vi "reshapeArray_FGV.vi"(4 "delete":dbl[](array[numeric])=[0.0, -1800.0, 0.0], 6 "firstpixelpos":dbl[](array[numeric]), 7 "command":T1=enum."read", 8 "error in (no error)":errorcluster, 9 "reshapedArray CamX":dbl[](array[numeric]), 10 "index":i32, 11 "emptyImageArray":dbl[](array[numeric])) -> (0 "error in (no error) 2":errorcluster, 3 "ImageArray":dbl[](array[numeric]))   [LabVIEW 2020]
uses:
  reshapeArrayCommand_TypDEf.ctl
panel:
  out "index 3":dbl
  out "del2 3":dbl
  out "del1 3":dbl
  out "size(s) 3":i32
  out "index 2":dbl
  out "del2 2":dbl
  out "del1 2":dbl
  out "size(s) 2":i32
  out "index":dbl
  out "Array":dbl[](array[numeric])
  in  "y":i32
  out "del2":dbl
  out "del1":dbl
  out "size(s)":i32
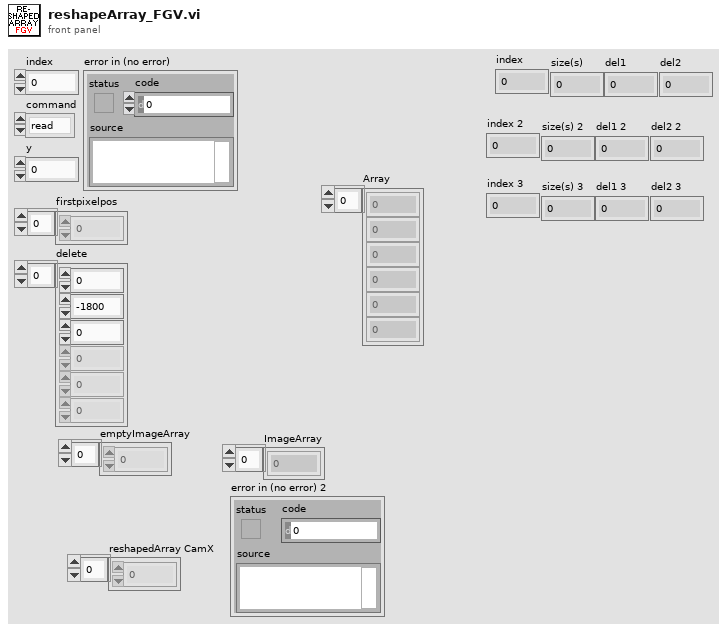
[diagram p1: front panel]
types:
  T1 = typedef "reshapeArrayCommand_TypDEf.ctl" = enum16{"init array", "addImage", "read", "init resolution"}
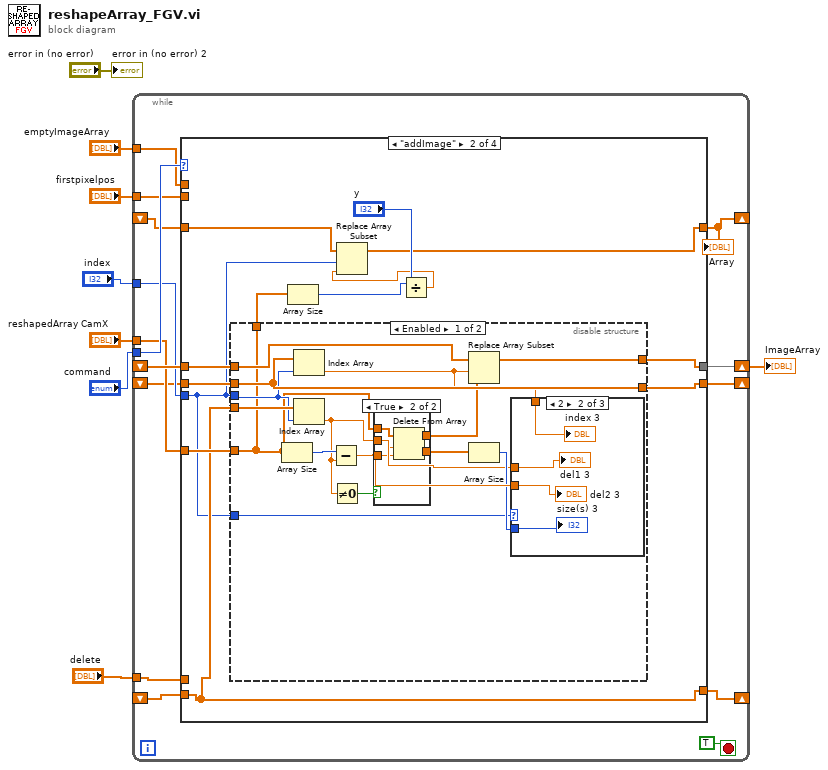
[diagram p0: block diagram]
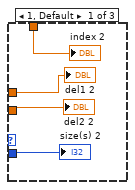
[diagram p4: hidden frame]
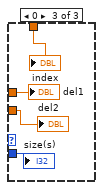
[diagram p5: hidden frame]
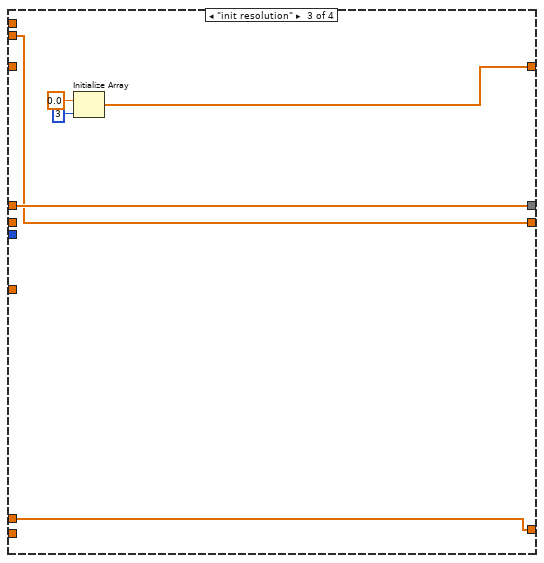
[diagram p7: hidden frame]
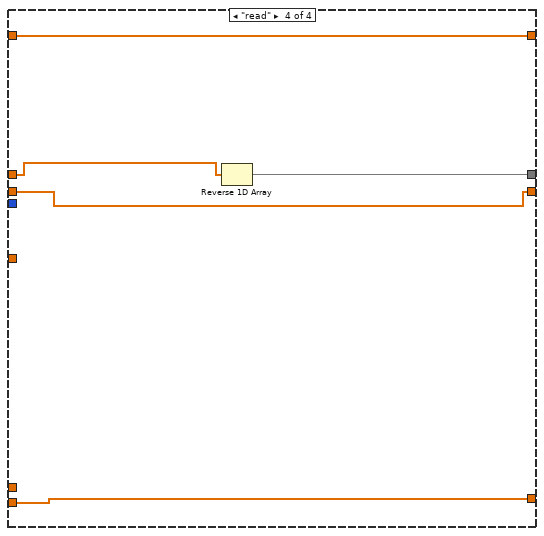
[diagram p8: hidden frame]
diagram:
  n1 = while {
    tunnel: "command" -> [w23]
    tunnel: "emptyImageArray" -> [w22]
    shift-right: [w21] -> w1
    shift-left: _ -> [w20]
    tunnel: "reshapedArray CamX" -> [w18]
    tunnel: "index" -> [w19]
    tunnel: "firstpixelpos" -> [w17]
    shift-right: [w15] -> _
    shift-left: _ -> [w14]
    tunnel: "delete" -> [w13]
    shift-right: [w12] -> _
    shift-left: _ -> [w11]
    shift-right: [w10] -> _
    shift-left: _ -> [w9]
    stop <- TRUE stop-if-true
    n2 = case shown="\"addImage\"" w23 {
      tunnel: w22 -> [w27 _ _ _]
      tunnel: [w27 w37 w79 w83] -> w21
      tunnel: w20 -> [_ w40 w79 w81]
      tunnel: w19 -> [_ w28 _ _]
      tunnel: w18 -> [_ w39 _ _]
      tunnel: w17 -> [_ _ w78 _]
      tunnel: [w26 w36 w78 w84] -> w15
      tunnel: w14 -> [w26 w38 _ w84]
      tunnel: w13 -> [_ _ w77 _]
      tunnel: [w25 w35 w77 w82] -> w12
      tunnel: w11 -> [w25 w35 _ w82]
      tunnel: [w24 w29 w74 w80] -> w10
      tunnel: w9 -> [w24 w30 _ w80]
      frame "init array", Default {
      }
      frame "addImage" {
        n3 = disable-structure shown="Enabled" {
          disable-tunnel: w40 -> [w51 _]
          disable-tunnel: w39 -> [w44 _]
          disable-tunnel: w28 -> [w52 _]
          disable-tunnel: w38 -> [w54 _]
          disable-tunnel: [w55 _] -> w37
          disable-tunnel: [w54 _] -> w36
          disable-tunnel: w35 -> [w53 _]
          disable-tunnel: [w44 _] -> w34
          disable-tunnel: w28 -> [w41 _]
          frame Enabled {
            n4 = Array Size(array=w44) -> (size(s)=w48:i32)
            n5 = Index Array(array=w54, index=w52) -> (element=w42:dbl)
            n6 = Index Array(array=w53, index=w52) -> (element=w43:dbl)
            n7 = Subtract(x=w48, y=w43) -> (x-y=w47:dbl)
            n8 = Not Equal To 0?(x=w43) -> (x != 0?=w45:bool)
            n9 = case shown="True" w45 {
              tunnel: [w56 w61] -> w50
              tunnel: [_ w60] -> w49
              tunnel: w44 -> [w56 w59]
              tunnel: w43 -> [_ w58]
              tunnel: w47 -> [_ w57]
              frame False {
              }
              frame True {
                n10 = Delete From Array(array=w59, length=w58, index=w57) -> (deleted portion=w60:dbl[], array with subset deleted=w61:dbl[])
              }
            }
            n11 = Replace Array Subset(array=w51, new element=w50, index=w42) -> (w55:dbl[])
            n12 = Array Size(array=w49) -> (size(s)=w46:i32)
            n13 = case shown="2" w41 {
              tunnel: w46 -> [w62 w69 w73]
              tunnel: w43 -> [w64 w67 w72]
              tunnel: w47 -> [w63 w68 w71]
              tunnel: w42 -> [w65 w66 w70]
              frame 1, Default {
                "del2 2" <- w63
                "del1 2" <- w64
                "index 2" <- w65
                "size(s) 2" <- w62
              }
              frame 2 {
                "del2 3" <- w68
                "del1 3" <- w67
                "index 3" <- w66
                "size(s) 3" <- w69
              }
              frame 0 {
                "size(s)" <- w73
                "del1" <- w72
                "del2" <- w71
                "index" <- w70
              }
            }
          }
          frame Disabled {
          }
        }
        n14 = Array Size(array=w34) -> (size(s)=w33:i32)
        n15 = Divide(x=w33, y="y") -> (x/y=w31:dbl)
        n16 = Replace Array Subset(array=w30, new element=w31, index=w28) -> (w29:dbl[])
      }
      frame "init resolution" {
        n17 = Initialize Array(0.0 ("element"), 3 ("dimension size")) -> (w74:dbl[])
      }
      frame "read" {
        n18 = Reverse 1D Array(array=w81) -> (reversed array=w83:dbl[])
      }
    }
    "Array" <- w10
  }
  "ImageArray" <- w1
  "error in (no error) 2" <- "error in (no error)"
